vi "AlgorithmLeftGoal2Copy.vi"(0 "MatchBallX":dbl, 1 "MatchBallY":dbl, 2 "D1 X COM":dbl, 3 "D1Y COM":dbl, 4 "D2 X COM":dbl, 5 "D2 Y COM":dbl) -> (9 "LW":T1, 11 "RW":cluster{"kRW":dbl, "CoRW":dbl, "y":dbl, "y":dbl}, 13 "output cluster":T2, 14 "Theta LG,LW":dbl, 15 "aRW":dbl, 16 "aS":dbl, 17 "min x":dbl, 18 "min x2":dbl, 19 "min x3":dbl)   [LabVIEW 2014]
panel:
  out "xD2BotS":dbl
  out "xD2ComS":dbl
  out "xD1BotS":dbl
  out "xD1ComS":dbl
  out "xD2BotR":dbl
  out "xD2ComR":dbl
  out "xD1BotR":dbl
  out "xD1ComR":dbl
  out "D2 X Bot fit 2":dbl
  out "D2 X Com fit":dbl
  out "D1 X Bot fit":dbl
  out "D1 X Com fit":dbl
  # "LOGIC"
  # "Left Goal"
  # "STRAIGHT"
  # "Left wall"
  # "Right Wall"
  # "Straight"
  # "sending data"
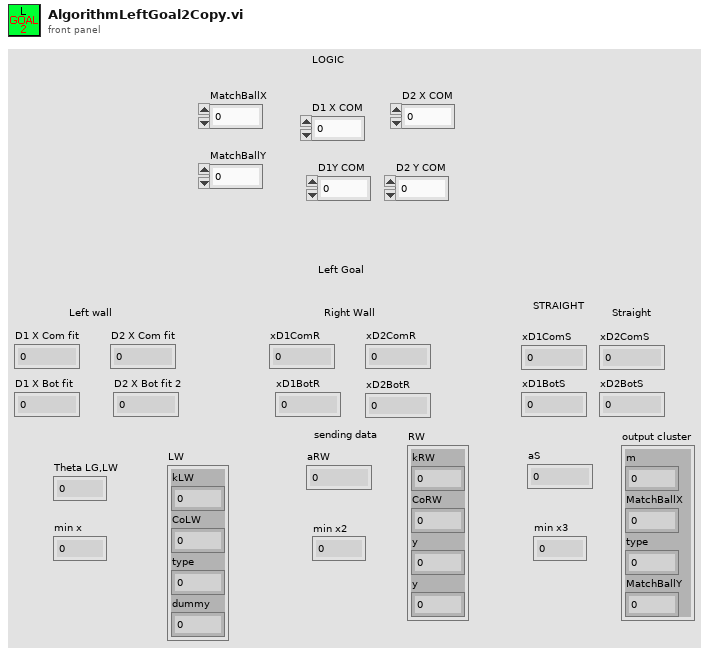
[diagram p1: front panel]
types:
  T1 = cluster{"kLW":dbl, "CoLW":dbl, "type":dbl, "dummy":dbl}
  T2 = cluster{"m":dbl, "MatchBallX":dbl, "type":dbl, "MatchBallY":dbl}
  T3 = cluster{"m":dbl, "MatchBallX":dbl, "y":dbl, "MatchBallY":dbl}
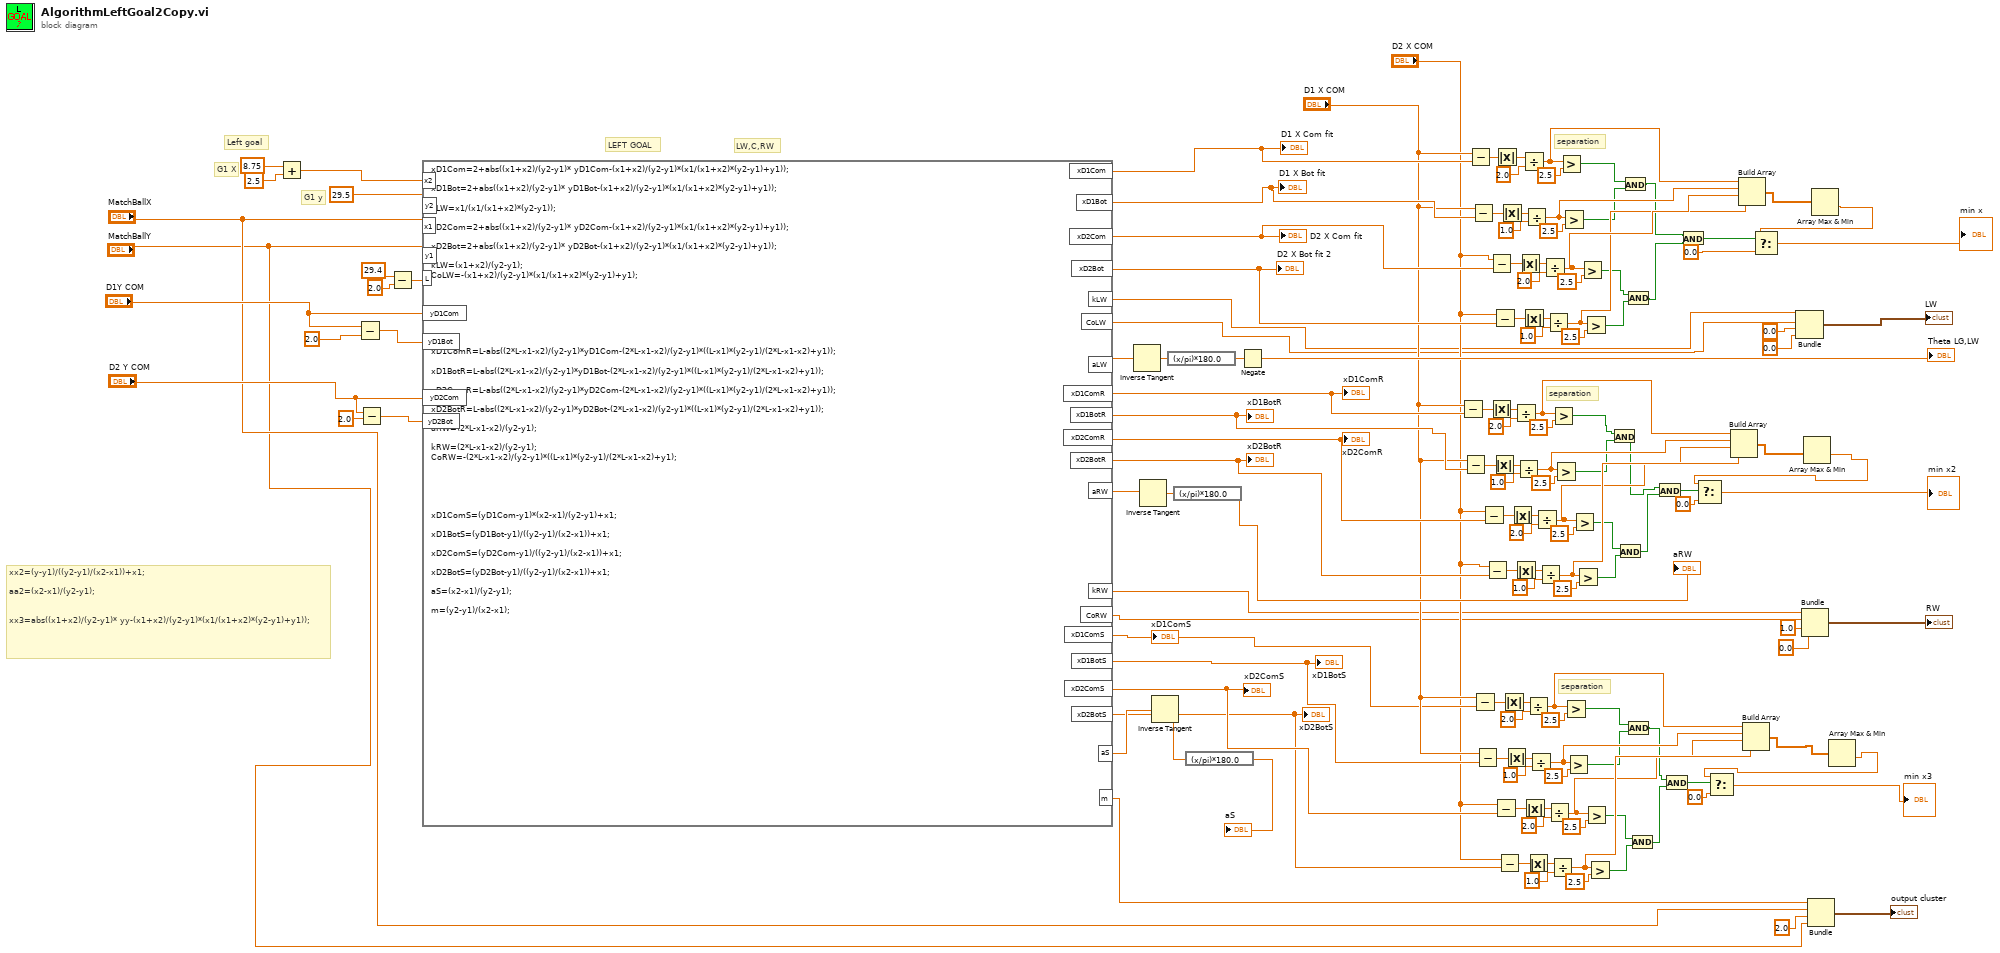
[diagram p0: block diagram]
diagram:
  # "LW,C,RW"
  # "separation"
  # "separation"
  # "separation"
  # "LEFT GOAL"
  # "xx2=(y-y1)/((y2-y1)/(x2-x1))+x1;\n\naa2=(x2-x1)/(y2-y1);\n\n\nxx3=abs((x1+x2)/(y2-y1)* yy-(x1+x2)/(y2-y1)*(x1/(x1+x2)*(y2-y1)+y1));"
  # "Left goal"
  # "G1 y"
  # "G1 X"
  n1 = Add(x=8.75, y=2.5) -> (x+y=w142:dbl)
  n2 = Subtract(x="D1Y COM", y=2.0) -> (x-y=w137:dbl)
  n3 = Subtract(x="D2 Y COM", y=2.0) -> (x-y=w132:dbl)
  n4 = Subtract(x=29.4 ("input variable"), y=2.0) -> (x-y=w17:dbl)
  n5 = formula code="xD1Com=2+abs((x1+x2)/(y2-y1)* yD1Com-(x1+x2)/(y2-y1)*(x1/(x1+x2)*(y2-y1)+y1));\n\nxD1Bot=2+abs((x1+x2)/(y2-y1)* yD1Bot-(x1+x2)/(y2-y1)*(x1/(x1+x2)*(y2-y1)+y1));\n\naLW=x1/(x1/(x1+x2)*(y2-y1));\n\nxD2Com=2+abs((x1+x2)/(y2-y1)* yD2Com-(x1+x2)/(y2-y1)*(x1/(x1+x2)*(y2-y1)+y1));\n\nxD2Bot=2+abs((x1+x2)/(y2-y1)* yD2Bot-(x1+x2)/(y2-y1)*(x1/(x1+x2)*(y2-y1)+y1));\n\nkLW=(x1+x2)/(y2-y1);\nCoLW=-(x1+x2)/(y2-y1)*(x1/(x1+x2)*(y2-y1)+y1);\n\n\n\n\n\n\n\nxD1ComR=L-abs((2*L-x1-x2)/(y2-y1)*yD1Com-(2*L-x1-x2)/(y2-y1)*((L-x1)*(y2-y1)/(2*L-x1-x2)+y1));\n\nxD1BotR=L-abs((2*L-x1-x2)/(y2-y1)*yD1Bot-(2*L-x1-x2)/(y2-y1)*((L-x1)*(y2-y1)/(2*L-x1-x2)+y1));\n\nxD2ComR=L-abs((2*L-x1-x2)/(y2-y1)*yD2Com-(2*L-x1-x2)/(y2-y1)*((L-x1)*(y2-y1)/(2*L-x1-x2)+y1));\n\nxD2BotR=L-abs((2*L-x1-x2)/(y2-y1)*yD2Bot-(2*L-x1-x2)/(y2-y1)*((L-x1)*(y2-y1)/(2*L-x1-x2)+y1));\n\naRW=(2*L-x1-x2)/(y2-y1);\n\nkRW=(2*L-x1-x2)/(y2-y1);\nCoRW=-(2*L-x1-x2)/(y2-y1)*((L-x1)*(y2-y1)/(2*L-x1-x2)+y1);\n\n\n\n\n\nxD1ComS=(yD1Com-y1)*(x2-x1)/(y2-y1)+x1;\n\nxD1BotS=(yD1Bot-y1)/((y2-y1)/(x2-x1))+x1;\n\nxD2ComS=(yD2Com-y1)/((y2-y1)/(x2-x1))+x1;\n\nxD2BotS=(yD2Bot-y1)/((y2-y1)/(x2-x1))+x1;\n\naS=(x2-x1)/(y2-y1);\n\nm=(y2-y1)/(x2-x1);"("x1"="MatchBallX", "x2"=w142, "y2"=29.5, "y1"="MatchBallY", "yD1Com"="D1Y COM", "yD2Com"="D2 Y COM", "yD1Bot"=w137, "yD2Bot"=w132, "L"=w17) -> ("xD1Com"=w125:dbl, "aLW"=w140:dbl, "xD1Bot"=w111:dbl, "xD2Com"=w116:dbl, "xD2Bot"=w106:dbl, "xD1ComR"=w79:dbl, "xD1BotR"=w78:dbl, "xD2ComR"=w77:dbl, "xD2BotR"=w76:dbl, "aRW"=w130:dbl, "xD1ComS"=w53:dbl, "aS"=w126:dbl, "xD1BotS"=w52:dbl, "xD2BotS"=w50:dbl, "xD2ComS"=w51:dbl, "kLW"=w15:dbl, "CoLW"=w14:dbl, "kRW"=w12:dbl, "CoRW"=w11:dbl, "m"=w9:dbl)
  "D1 X Com fit" <- w125
  "D1 X Bot fit" <- w111
  "D2 X Com fit" <- w116
  "D2 X Bot fit 2" <- w106
  "xD1ComR" <- w79
  "xD1BotR" <- w78
  "xD2ComR" <- w77
  "xD2BotR" <- w76
  "xD1ComS" <- w53
  "xD1BotS" <- w52
  "xD2ComS" <- w51
  "xD2BotS" <- w50
  n6 = Inverse Tangent(1:w140) -> (0:w141:dbl)
  n7 = Inverse Tangent(1:w130) -> (0:w131:dbl)
  n8 = Inverse Tangent(1:w126) -> (0:w127:dbl)
  n9 = expression code="(x/pi)*180.0" ("radians to degrees")(w141) -> (w138:dbl)
  n10 = expression code="(x/pi)*180.0" ("radians to degrees")(w131) -> (→"aRW":dbl)
  n11 = expression code="(x/pi)*180.0" ("radians to degrees")(w127) -> (→"aS":dbl)
  n12 = Negate(x=w138) -> (-x=→"Theta LG,LW":dbl)
  n13 = Subtract(x="D1 X COM", y=w79) -> (x-y=w80:dbl)
  n14 = Subtract(x="D1 X COM", y=w78) -> (x-y=w91:dbl)
  n15 = Subtract(x="D1 X COM", y=w125) -> (x-y=w124:dbl)
  n16 = Subtract(x="D1 X COM", y=w111) -> (x-y=w112:dbl)
  n17 = Subtract(x="D1 X COM", y=w53) -> (x-y=w55:dbl)
  n18 = Subtract(x="D1 X COM", y=w52) -> (x-y=w66:dbl)
  n19 = Subtract(x="D2 X COM", y=w77) -> (x-y=w87:dbl)
  n20 = Subtract(x="D2 X COM", y=w76) -> (x-y=w92:dbl)
  n21 = Subtract(x="D2 X COM", y=w116) -> (x-y=w117:dbl)
  n22 = Absolute Value(x=w80) -> (abs(x)=w81:dbl)
  n23 = Absolute Value(x=w91) -> (abs(x)=w90:dbl)
  n24 = Subtract(x="D2 X COM", y=w106) -> (x-y=w110:dbl)
  n25 = Subtract(x="D2 X COM", y=w51) -> (x-y=w62:dbl)
  n26 = Absolute Value(x=w124) -> (abs(x)=w123:dbl)
  n27 = Subtract(x="D2 X COM", y=w50) -> (x-y=w67:dbl)
  n28 = Absolute Value(x=w112) -> (abs(x)=w113:dbl)
  n29 = Absolute Value(x=w55) -> (abs(x)=w56:dbl)
  n30 = Absolute Value(x=w66) -> (abs(x)=w65:dbl)
  n31 = Absolute Value(x=w87) -> (abs(x)=w86:dbl)
  n32 = Divide(x=w81, y=2.0) -> (x/y=w97:dbl)
  n33 = Absolute Value(x=w92) -> (abs(x)=w93:dbl)
  n34 = Divide(x=w90, y=1.0) -> (x/y=w98:dbl)
  n35 = Absolute Value(x=w117) -> (abs(x)=w118:dbl)
  n36 = Divide(x=w123, y=2.0) -> (x/y=w104:dbl)
  n37 = Absolute Value(x=w110) -> (abs(x)=w109:dbl)
  n38 = Absolute Value(x=w62) -> (abs(x)=w61:dbl)
  n39 = Divide(x=w113, y=1.0) -> (x/y=w103:dbl)
  n40 = Divide(x=w56, y=2.0) -> (x/y=w72:dbl)
  n41 = Absolute Value(x=w67) -> (abs(x)=w68:dbl)
  n42 = Divide(x=w65, y=1.0) -> (x/y=w73:dbl)
  n43 = Divide(x=w86, y=2.0) -> (x/y=w99:dbl)
  n44 = Divide(x=w93, y=1.0) -> (x/y=w100:dbl)
  n45 = Divide(x=w118, y=2.0) -> (x/y=w102:dbl)
  n46 = Divide(x=w109, y=1.0) -> (x/y=w101:dbl)
  n47 = Divide(x=w61, y=2.0) -> (x/y=w74:dbl)
  n48 = Divide(x=w68, y=1.0) -> (x/y=w75:dbl)
  n49 = Greater?(x=w97, y=2.5) -> (0:w36:bool)
  n50 = Greater?(x=w98, y=2.5) -> (0:w35:bool)
  n51 = Greater?(x=w104, y=2.5) -> (0:w41:bool)
  n52 = Greater?(x=w103, y=2.5) -> (0:w40:bool)
  n53 = Greater?(x=w72, y=2.5) -> (0:w31:bool)
  n54 = Greater?(x=w73, y=2.5) -> (0:w30:bool)
  n55 = Greater?(x=w99, y=2.5) -> (0:w34:bool)
  n56 = Greater?(x=w100, y=2.5) -> (0:w33:bool)
  n57 = Greater?(x=w102, y=2.5) -> (0:w45:bool)
  n58 = Greater?(x=w101, y=2.5) -> (0:w44:bool)
  n59 = Greater?(x=w74, y=2.5) -> (0:w28:bool)
  n60 = Greater?(x=w75, y=2.5) -> (0:w27:bool)
  n61 = And(x=w36, y=w35) -> (x .and. y?=w37:bool)
  n62 = And(x=w34, y=w33) -> (x .and. y?=w32:bool)
  n63 = And(x=w41, y=w40) -> (x .and. y?=w39:bool)
  n64 = And(x=w45, y=w44) -> (x .and. y?=w42:bool)
  n65 = And(x=w31, y=w30) -> (x .and. y?=w29:bool)
  n66 = And(x=w28, y=w27) -> (x .and. y?=w26:bool)
  n67 = And(x=w37, y=w32) -> (x .and. y?=w38:bool)
  n68 = And(x=w29, y=w26) -> (x .and. y?=w25:bool)
  n69 = And(x=w39, y=w42) -> (x .and. y?=w43:bool)
  n70 = Build Array(w97, w98, w99, w100) -> (w22:dbl[])
  n71 = Build Array(w104, w103, w102, w101) -> (w24:dbl[])
  n72 = Build Array(w72, w73, w74, w75) -> (w20:dbl[])
  n73 = Bundle("kLW"=w15, "CoLW"=w14, "y"=0.0, "y"=0.0) -> (→"LW":cluster{"kLW":dbl, "CoLW":dbl, "y":dbl, "y":dbl})  [unwired: 1 in]
  n74 = Bundle("kRW"=w12, "CoRW"=w11, "y"=1.0, "y"=0.0) -> (→"RW":cluster{"kRW":dbl, "CoRW":dbl, "y":dbl, "y":dbl})  [unwired: 1 in]
  n75 = Array Max & Min(array=w22) -> (min value=w21:dbl)  [unwired: 3 out]
  n76 = Select(t=w21, s=w38, f=0.0 ("y")) -> (s? t:f=→"min x2":dbl)
  n77 = Bundle("m"=w9, "MatchBallX"="MatchBallX", "y"=2.0, "MatchBallY"="MatchBallY") -> (→"output cluster":T3)  [unwired: 1 in]
  n78 = Array Max & Min(array=w24) -> (min value=w23:dbl)  [unwired: 3 out]
  n79 = Select(t=w23, s=w43, f=0.0 ("y")) -> (s? t:f=→"min x":dbl)
  n80 = Array Max & Min(array=w20) -> (min value=w19:dbl)  [unwired: 3 out]
  n81 = Select(t=w19, s=w25, f=0.0 ("y")) -> (s? t:f=→"min x3":dbl)
